vi "1553B_帧解析_字符串_v4_21.vi"(11 "输入簇":T1) -> (2 "脉冲数":string, 3 "温度":string)   [LabVIEW 2012]
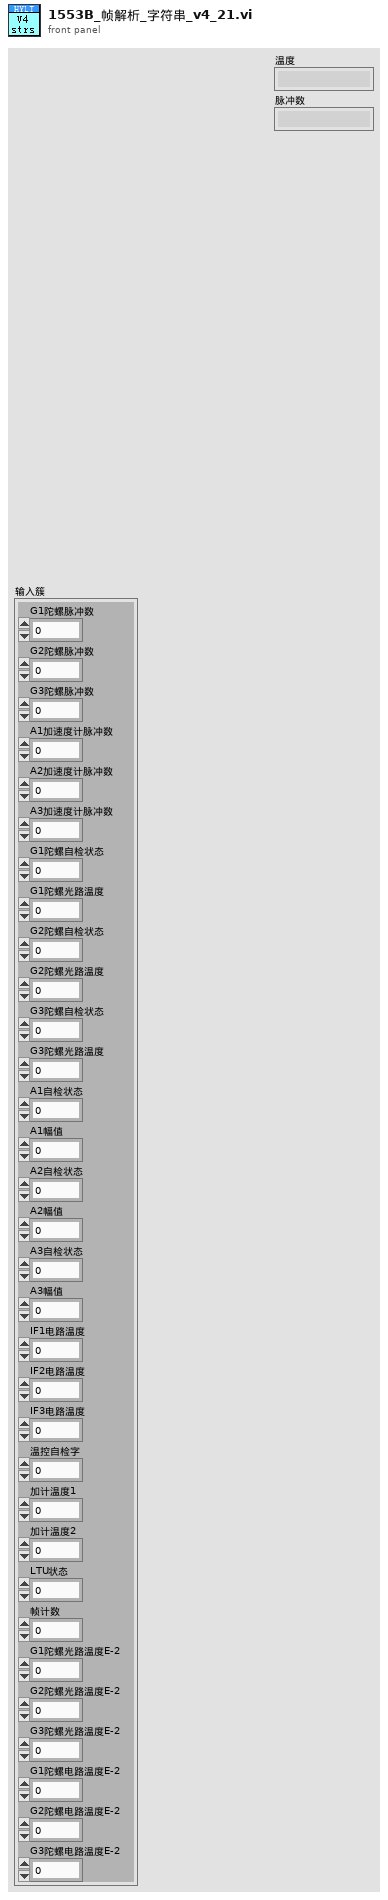
[diagram p1: front panel]
types:
  T1 = cluster{"G1陀螺脉冲数":i32, "G2陀螺脉冲数":i32, "G3陀螺脉冲数":i32, "A1加速度计脉冲数":i16, "A2加速度计脉冲数":i16, "A3加速度计脉冲数":i16, "G1陀螺自检状态":u8, "G1陀螺光路温度":i8, "G2陀螺自检状态":u8, "G2陀螺光路温度":i8, "G3陀螺自检状态":u8, "G3陀螺光路温度":i8, "A1自检状态":u8, "A1幅值":u8, "A2自检状态":u8, "A2幅值":u8, "A3自检状态":u8, "A3幅值":u8, "IF1电路温度":i8, "IF2电路温度":i8, "IF3电路温度":i8, "温控自检字":u8, "加计温度1":i16, "加计温度2":i16, "LTU状态":u8, "帧计数":u8, "G1陀螺光路温度E-2":i16, "G2陀螺光路温度E-2":i16, "G3陀螺光路温度E-2":i16, "G1陀螺电路温度E-2":i16, "G2陀螺电路温度E-2":i16, "G3陀螺电路温度E-2":i16}
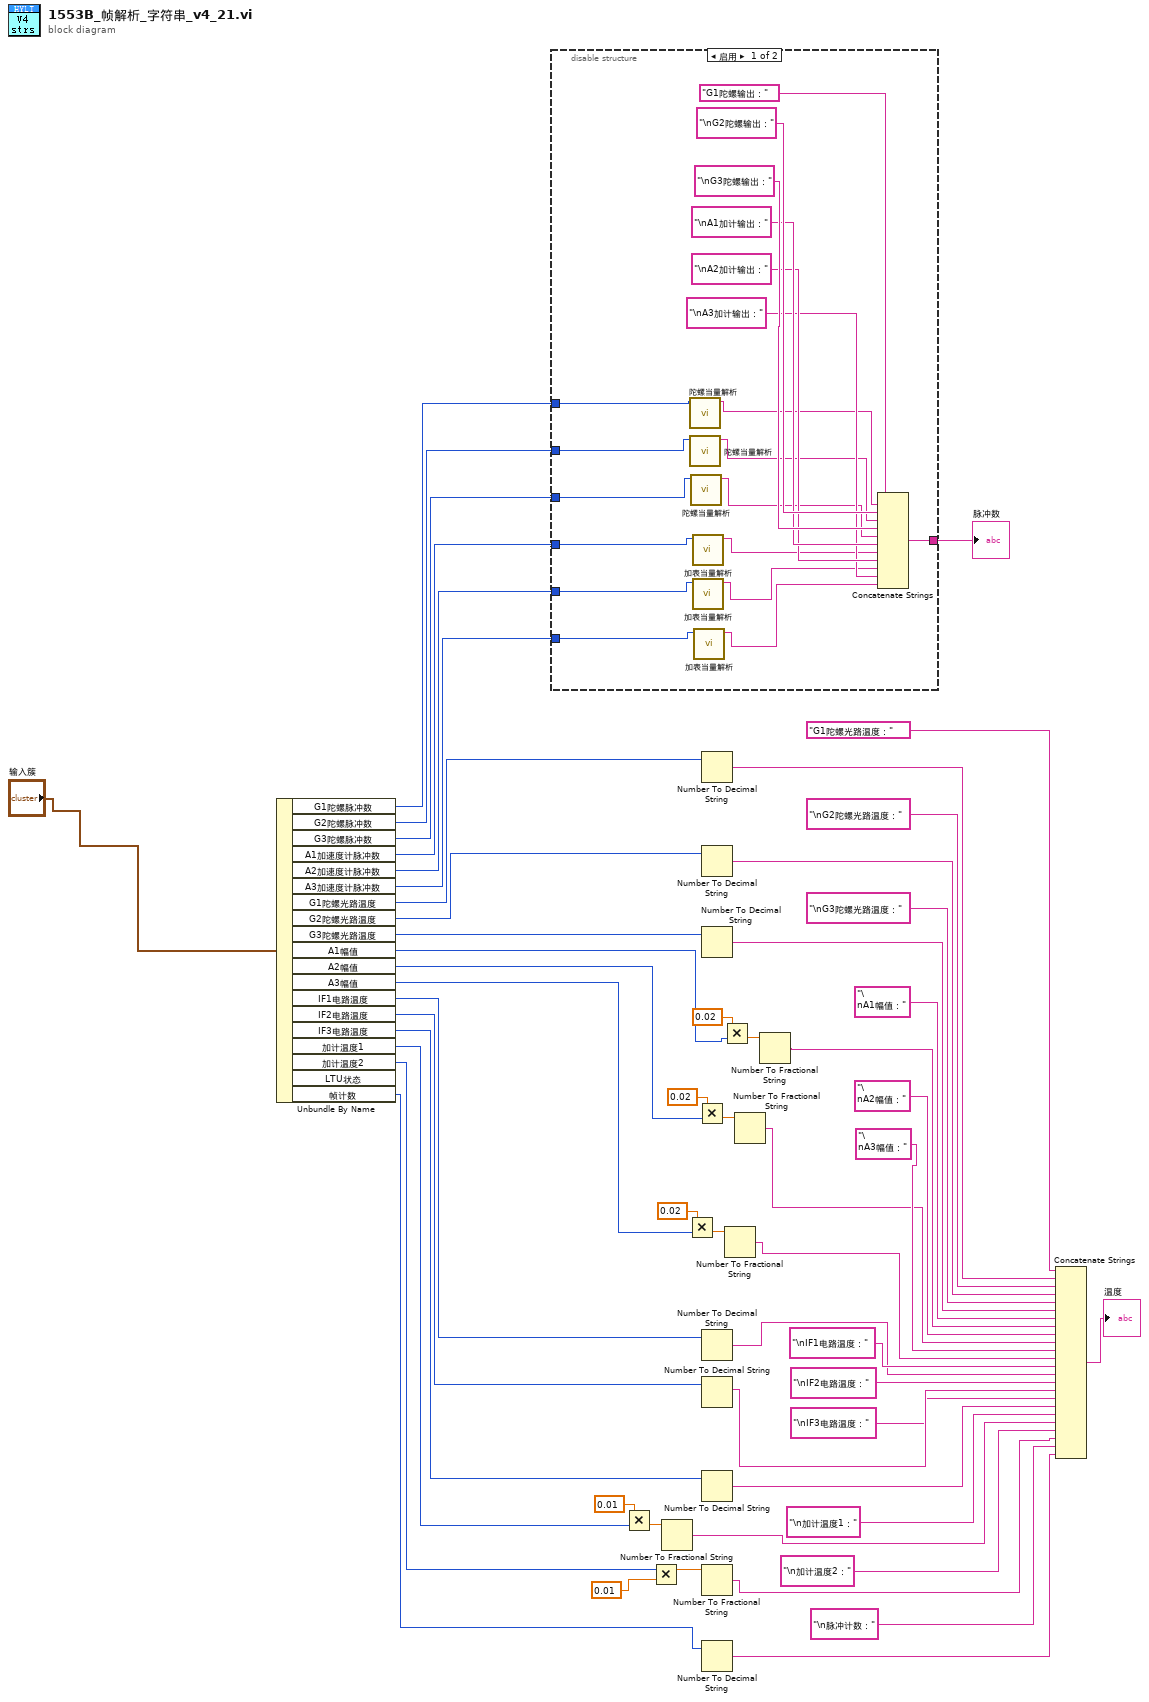
[diagram p0: block diagram]
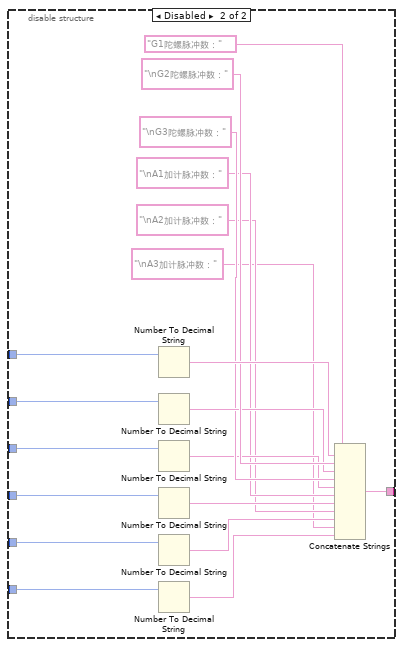
[diagram p2: hidden frame]
diagram:
  n1 = Unbundle By Name("输入簇") -> ("G1陀螺脉冲数"=w53:i32, "G2陀螺脉冲数"=w52:i32, "G3陀螺脉冲数"=w51:i32, "A1加速度计脉冲数"=w50:i16, "A2加速度计脉冲数"=w55:i16, "A3加速度计脉冲数"=w54:i16, "G1陀螺光路温度"=w41:i8, "G2陀螺光路温度"=w40:i8, "G3陀螺光路温度"=w39:i8, "A1幅值"=w5:u8, "A2幅值"=w1:u8, "A3幅值"=w4:u8, "IF1电路温度"=w36:i8, "IF2电路温度"=w35:i8, "IF3电路温度"=w34:i8, "加计温度1"=w25:i16, "加计温度2"=w24:i16, "帧计数"=w20:u8)  [unwired: 1 out]
  n2 = disable-structure shown="启用" {
    disable-tunnel: w55 -> [w60 w93]
    disable-tunnel: w54 -> [w59 w92]
    disable-tunnel: w53 -> [w66 w79]
    disable-tunnel: w52 -> [w65 w78]
    disable-tunnel: w51 -> [w63 w77]
    disable-tunnel: w50 -> [w61 w76]
    disable-tunnel: [w68 w75] -> w37
    frame Enabled {
      n3 = call "陀螺当量解析.vi"("输入"=w66) -> ("输出"=w67:string)  [unwired: 9 in, 1 out]
      n4 = call "陀螺当量解析.vi"("输入"=w65) -> ("输出"=w64:string)  [unwired: 9 in, 1 out]
      n5 = call "陀螺当量解析.vi"("输入"=w63) -> ("输出"=w62:string)  [unwired: 9 in, 1 out]
      n6 = call "加表当量解析.vi"("输入"=w61) -> ("输出"=w56:string)  [unwired: 9 in, 1 out]
      n7 = call "加表当量解析.vi"("输入"=w60) -> ("输出"=w57:string)  [unwired: 9 in, 1 out]
      n8 = call "加表当量解析.vi"("输入"=w59) -> ("输出"=w58:string)  [unwired: 9 in, 1 out]
      n9 = Concatenate Strings("G1陀螺输出：" ("字符串"), w67, "\nG2陀螺输出：" ("字符串"), w64, "\nG3陀螺输出：" ("字符串"), w62, "\nA1加计输出：" ("字符串"), w56, "\nA2加计输出：" ("字符串"), w57, "\nA3加计输出：" ("字符串"), w58) -> (w68:string)
    }
    frame Disabled {
      n10 = Number To Decimal String(number=w79) -> (decimal integer string=w90:string)  [unwired: 1 in]
      n11 = Number To Decimal String(number=w78) -> (decimal integer string=w88:string)  [unwired: 1 in]
      n12 = Number To Decimal String(number=w77) -> (decimal integer string=w86:string)  [unwired: 1 in]
      n13 = Number To Decimal String(number=w76) -> (decimal integer string=w84:string)  [unwired: 1 in]
      n14 = Number To Decimal String(number=w93) -> (decimal integer string=w82:string)  [unwired: 1 in]
      n15 = Number To Decimal String(number=w92) -> (decimal integer string=w80:string)  [unwired: 1 in]
      n16 = Concatenate Strings("G1陀螺脉冲数：" ("字符串"), w90, "\nG2陀螺脉冲数：" ("字符串"), w88, "\nG3陀螺脉冲数：" ("字符串"), w86, "\nA1加计脉冲数：" ("字符串"), w84, "\nA2加计脉冲数：" ("字符串"), w82, "\nA3加计脉冲数：" ("字符串"), w80) -> (w75:string)
    }
  }
  "脉冲数" <- w37
  n17 = Multiply(x=0.01, y=w25) -> (x*y=w16:dbl)
  n18 = Multiply(x=w24, y=0.01) -> (x*y=w14:dbl)
  n19 = Number To Fractional String(number=w16) -> (F-format string=w15:string)  [unwired: 3 in]
  n20 = Multiply(x=0.02, y=w4) -> (x*y=w11:dbl)
  n21 = Multiply(x=0.02, y=w1) -> (x*y=w9:dbl)
  n22 = Number To Decimal String(number=w41) -> (decimal integer string=w43:string)  [unwired: 1 in]
  n23 = Number To Decimal String(number=w40) -> (decimal integer string=w45:string)  [unwired: 1 in]
  n24 = Number To Decimal String(number=w39) -> (decimal integer string=w47:string)  [unwired: 1 in]
  n25 = Number To Decimal String(number=w36) -> (decimal integer string=w30:string)  [unwired: 1 in]
  n26 = Number To Decimal String(number=w35) -> (decimal integer string=w28:string)  [unwired: 1 in]
  n27 = Number To Decimal String(number=w34) -> (decimal integer string=w26:string)  [unwired: 1 in]
  n28 = Number To Fractional String(number=w14) -> (F-format string=w21:string)  [unwired: 3 in]
  n29 = Number To Decimal String(number=w20) -> (decimal integer string=w19:string)  [unwired: 1 in]
  n30 = Multiply(x=0.02, y=w5) -> (x*y=w7:dbl)
  n31 = Number To Fractional String(number=w11) -> (F-format string=w3:string)  [unwired: 3 in]
  n32 = Number To Fractional String(number=w9) -> (F-format string=w2:string)  [unwired: 3 in]
  n33 = Number To Fractional String(number=w7) -> (F-format string=w6:string)  [unwired: 3 in]
  n34 = Concatenate Strings("G1陀螺光路温度：" ("字符串"), w43, "\nG2陀螺光路温度：" ("字符串"), w45, "\nG3陀螺光路温度：" ("字符串"), w47, "\nA1幅值：" ("字符串"), w6, "\nA2幅值：" ("字符串"), w2, "\nA3幅值：" ("字符串"), w3, "\nIF1电路温度：" ("字符串"), w30, "\nIF2电路温度：" ("字符串"), w28, "\nIF3电路温度：" ("字符串"), w26, "\n加计温度1：" ("字符串"), w15, "\n加计温度2：" ("字符串"), w21, "\n脉冲计数：" ("字符串"), w19) -> (→"温度":string)
